vi "subSave_DaqData.vi"(5 "Waveform type (complete)":u16(ring) items=["Complete waveforms", "Analog In only", "Optopatch"], 7 "path":path, 8 "Camera in (no error)":errorcluster, 9 "Test Patch array":dbl[](array[numeric]), 10 "AI waveform":dbl[][](graph), 11 "DI waveform":digitalwaveform(graph)) -> (0 "Camera out":errorcluster)   [LabVIEW 2015]
uses:
  <vilib>/Waveform/DWDTOps.llb/DWDT Digital to Boolean Array.vi
  <vilib>/Utility/file.llb/Write Delimited Spreadsheet (string).vi
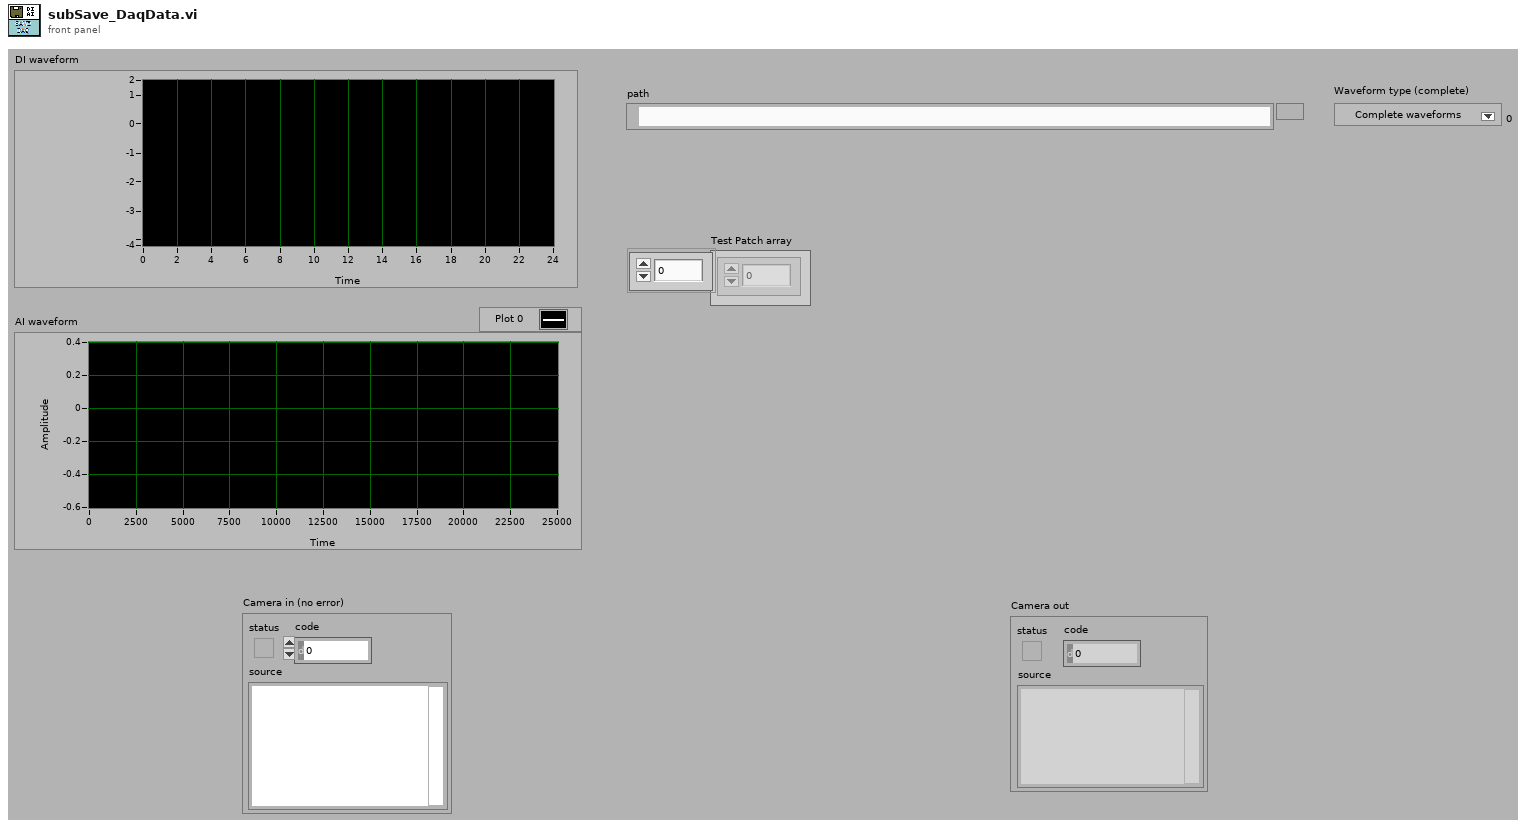
[diagram p1: front panel]
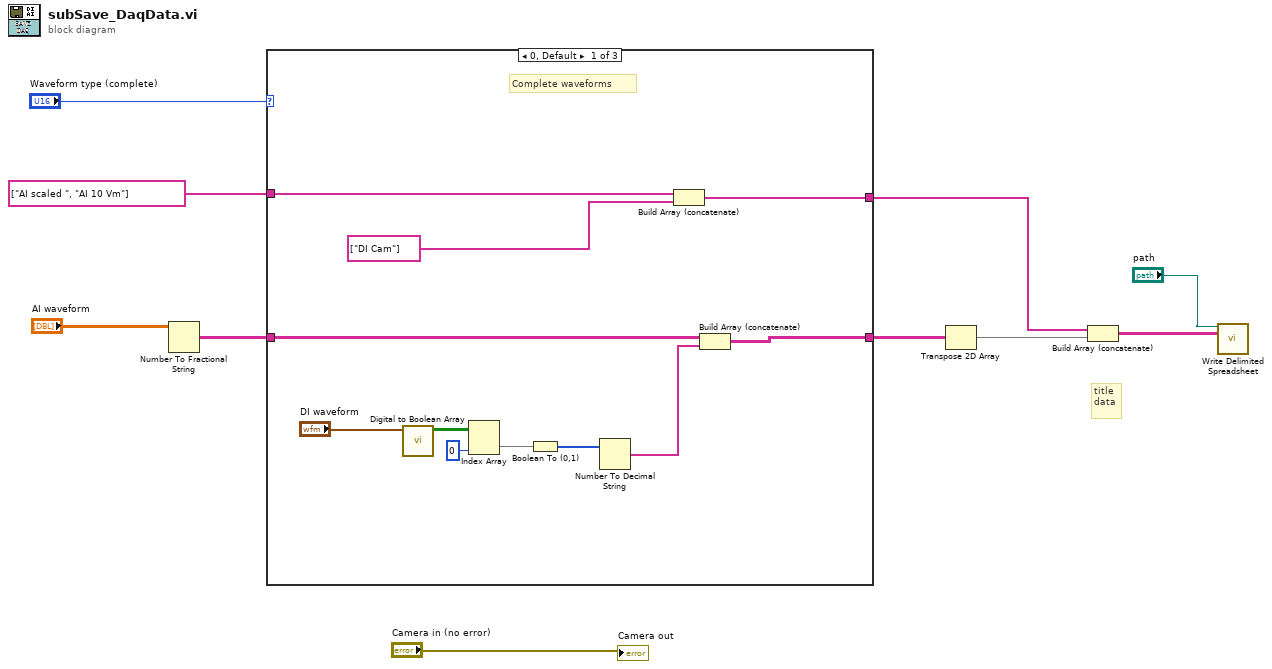
[diagram p0: block diagram]
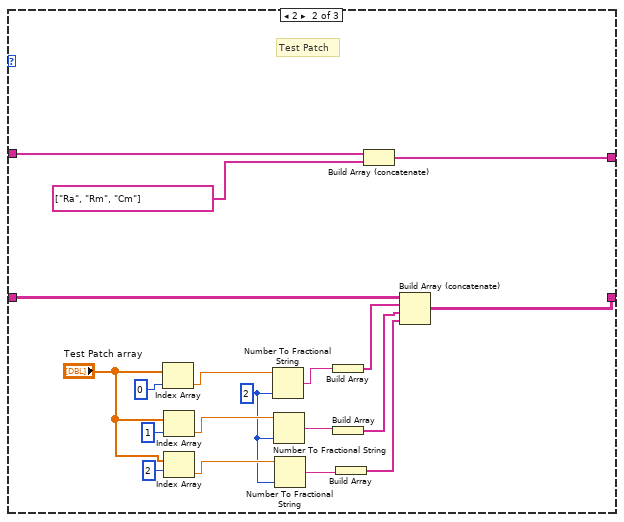
[diagram p2: hidden frame]
diagram:
  # "title\ndata"
  n1 = Number To Fractional String(number="AI waveform") -> (F-format string=w4:string[][])  [unwired: 3 in]
  n2 = case shown="0, Default" "Waveform type (complete)" {
    tunnel: [w19 w38 w42] -> w7
    tunnel: string[] ["AI scaled ", "AI 10 Vm"] -> [w21 w39 w42]
    tunnel: [w17 w36 w41] -> w3
    tunnel: w4 -> [w18 w37 w41]
    frame 0, Default {
      # "Complete waveforms"
      n3 = call-poly <vilib>:"Digital to Boolean Array.vi"("digital waveform"="DI waveform") -> ("boolean array"=w13:bool[][])  [unwired: 9 in, 1 out]
      n4 = Index Array(array=w13, index (col)=0 ("disabled index (col)")) -> (element=w15:bool[])  [unwired: 1 in]
      n5 = Boolean To (0,1)(Boolean=w15) -> (0, 1=w16:i16[])
      n6 = Number To Decimal String(number=w16) -> (decimal integer string=w11:string[])  [unwired: 1 in]
      n7 = Build Array (concatenate)(w21, string[] ["DI Cam"]) -> (w19:string[])
      n8 = Build Array (concatenate)(w18, w11) -> (w17:string[][])
    }
    frame 2 {
      w22 = i16 2 ("precision (6)")
      # "Test Patch"
      n9 = Index Array(array="Test Patch array", index=0) -> (element=w35:dbl)
      n10 = Index Array(array="Test Patch array", index=1) -> (element=w30:dbl)
      n11 = Index Array(array="Test Patch array", index=2) -> (element=w29:dbl)
      n12 = Number To Fractional String(number=w35, precision (6)=w22) -> (F-format string=w27:string)  [unwired: 2 in]
      n13 = Number To Fractional String(number=w30, precision (6)=w22) -> (F-format string=w26:string)  [unwired: 2 in]
      n14 = Number To Fractional String(number=w29, precision (6)=w22) -> (F-format string=w24:string)  [unwired: 2 in]
      n15 = Build Array(w27) -> (w28:string[])
      n16 = Build Array(w26) -> (w25:string[])
      n17 = Build Array(w24) -> (w23:string[])
      n18 = Build Array (concatenate)(w39, string[] ["Ra", "Rm", "Cm"]) -> (w38:string[])
      n19 = Build Array (concatenate)(w37, w28, w25, w23) -> (w36:string[][])
    }
    frame 1 {
      # "AI only"
    }
  }
  n20 = Transpose 2D Array(2D array=w3) -> (transposed array=w10:string[][])
  n21 = Build Array (concatenate)(w7, w10) -> (w2:string[][])
  n22 = call-poly <vilib>:"Write Delimited Spreadsheet.vi"("file path (dialog if empty)"="path", "2D data"=w2) -> ()  [unwired: 12 in, 2 out]
  "Camera out" <- "Camera in (no error)"
